vi "_Destroy.vi"(8 "error in (no error)":errorcluster, 11 "Photon Counter SR400 in":refnum<class "Photon Counter SR400.lvclass">) -> (0 "error out":errorcluster)   [LabVIEW 2017, in "Photon Counter SR400.lvclass"]
uses:
  Photon Counter SR400.lvclass
  Utility Classes/Readable/Readable.lvclass
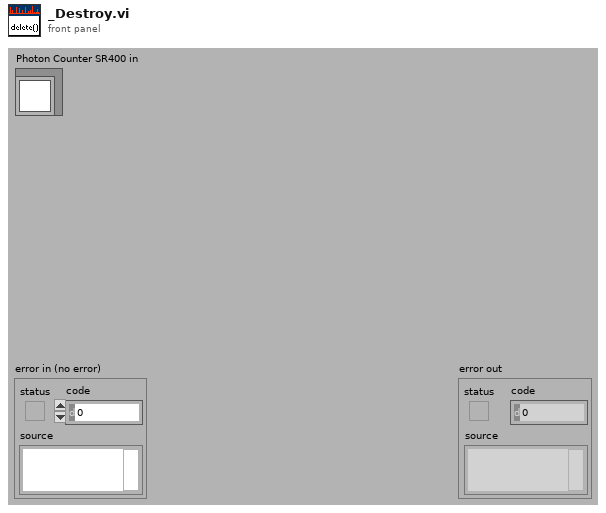
[diagram p1: front panel]
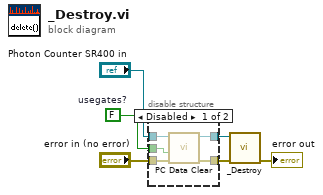
[diagram p0: block diagram]
diagram:
  w3 = FALSE  # usegates?
  n1 = disable-structure shown="Disabled" {
    disable-tunnel: "error in (no error)" -> [w11 w12]
    disable-tunnel: [w10 w12] -> w4
    disable-tunnel: w3 -> [w9 _]
    disable-tunnel: "Photon Counter SR400 in" -> [w8 w13]
    disable-tunnel: [w7 w13] -> w1
    frame Disabled {
      n2 = call "PC Data Clear.vi"("errorIN"=w11, "usegates?"=w9, "Photon Counter SR400 in"=w8) -> ("errorOUT"=w10:errorcluster, "Photon Counter SR400 out"=w7:refnum<class "Photon Counter SR400.lvclass">)  [unwired: 1 in, 6 out]
    }
    frame Enabled {
    }
  }
  n3 = call-parent "_Destroy.vi"("error in (no error)"=w4, "Instrument in"=w1) -> ("error out"=→"error out":errorcluster)  [unwired: 9 out]
